vi "main.vi"() -> ()   [LabVIEW 2021]
uses:
  CTLs/msg.ctl
  <vilib>/MakerHub/LINX/Private/Type Defs/LINX Ref.ctl
  <vilib>/MakerHub/LINX/Private/Type Defs/Platform.ctl
  <vilib>/MakerHub/LINX/Private/Type Defs/Interface.ctl
  <vilib>/MakerHub/LINX/Private/Device/Type Defs/LINX Device Config.ctl
  <vilib>/MakerHub/LINX/Private/Device/Type Defs/TCP Config.ctl
  <vilib>/MakerHub/LINX/Private/Device/Type Defs/Channels.ctl
  <vilib>/MakerHub/LINX/Private/Local IO/LinxI2cWrite.vi
  <vilib>/MakerHub/LINX/Public/Utilities/Check Channel.vi
  <vilib>/MakerHub/LINX/Public/Utilities/Open Serial.vi
  <vilib>/MakerHub/LINX/Private/Utilties/Generate Error.vi
  <vilib>/Utility/error.llb/Error Cluster From Error Code.vi
  <vilib>/ErrorRing/Error Ring.xnode
  <vilib>/MakerHub/LINX/LMH-LINX.lvlib
  <vilib>/MakerHub/LINX/Private/Device/Device.lvlib
panel:
  in  "info.I2C Slave Address":u8
  in  "info.Data":u8[](array[numeric])
  in  "Serial Port":refnum<visa-resource-name>="N/A"
  in  "Error In":errorcluster
  in  "error in (no error)":errorcluster
  in  "msg":T1={"mensaje"="", "info"={"I2C Slave Address "=0, "Data"=[0]}, "LINX Resource"={"IO"=enum."Remote", "Interface"=enum."Serial", "LINX Device Config"={"Interface"=enum."Serial", "COM Port"="", "TCP Configuration"={"IP Address"="", "Port"=0}, "Device Family"=0, "Device ID"=0, "Device Name"="", "TCP Ref"=refnum, "Channels"={"DI"=[], "DO"=[], "AI"=[], "AO"=[], "PWM"=[], "QE"=[], "UART"=[], "I2C 2"=[], "SPI"=[], "CAN"=[], "Servo"=[], "AI Ref (V)"=0.0, "AI Resolution (Bits)"=0, "AO Ref (V)"=0.0, "AO Resolution (Bits)"=0}}}}
  in  "Stop":bool
  in  "Action 2":bool
  in  "Escribir":bool
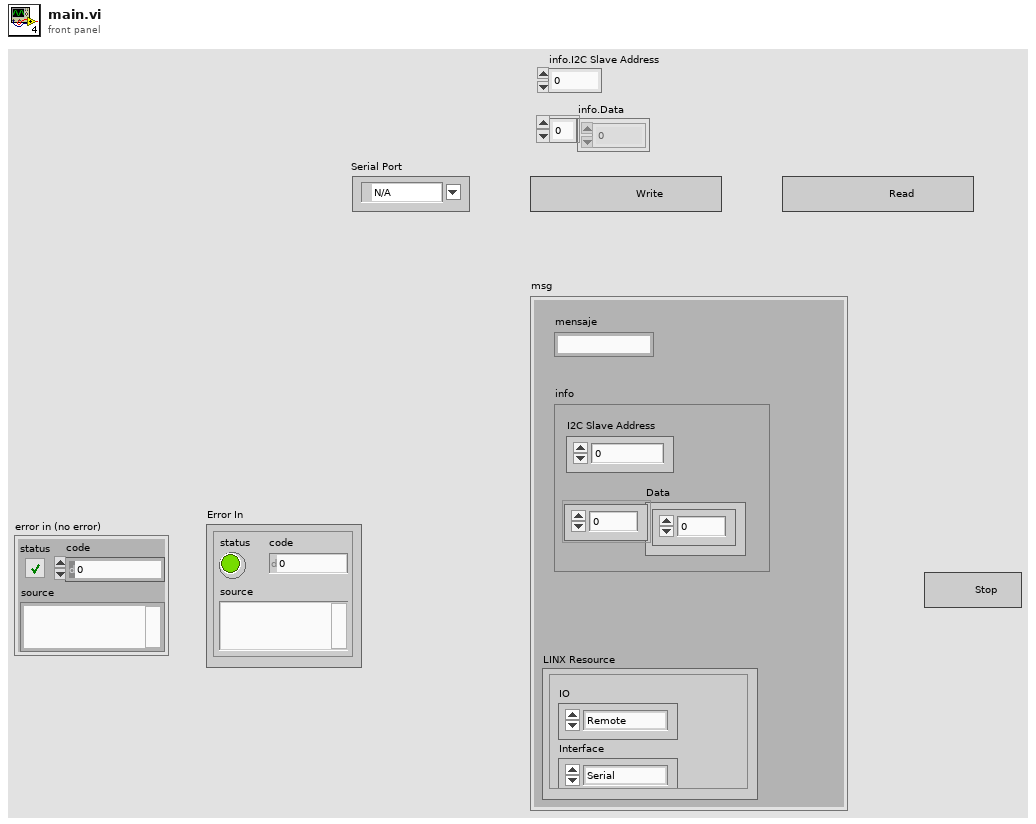
[diagram p1: front panel]
types:
  T1 = typedef "msg.ctl" = cluster{"mensaje":string, "info":cluster{"I2C Slave Address ":u8, "Data":u8[]}, "LINX Resource":T2}
  T2 = typedef "LMH-LINX.lvlib/LINX Ref.ctl" = cluster{"IO":T3, "Interface":T4, "LINX Device Config":T5}
  T3 = typedef "LMH-LINX.lvlib/Platform.ctl" = enum16{"Remote", "Local"}
  T4 = typedef "LMH-LINX.lvlib/Interface.ctl" = enum16{"Serial", "TCP"}
  T5 = typedef "LMH-LINX.lvlib/Device.lvlib/LINX Device Config.ctl" = cluster{"Interface":T4, "COM Port":refnum<visa-resource-name>, "TCP Configuration":T6, "Device Family":u8, "Device ID":u8, "Device Name":string, "TCP Ref":refnum<k5>, "Channels":T7}
  T6 = typedef "LMH-LINX.lvlib/Device.lvlib/TCP Config.ctl" = cluster{"IP Address":string, "Port":u16}
  T7 = typedef "LMH-LINX.lvlib/Channels.ctl" = cluster{"DI":u8[], "DO":u8[], "AI":u8[], "AO":u8[], "PWM":u8[], "QE":u8[], "UART":u8[], "I2C 2":u8[], "SPI":u8[], "CAN":u8[], "Servo":u8[], "AI Ref (V)":dbl, "AI Resolution (Bits)":u8, "AO Ref (V)":dbl, "AO Resolution (Bits)":u8}
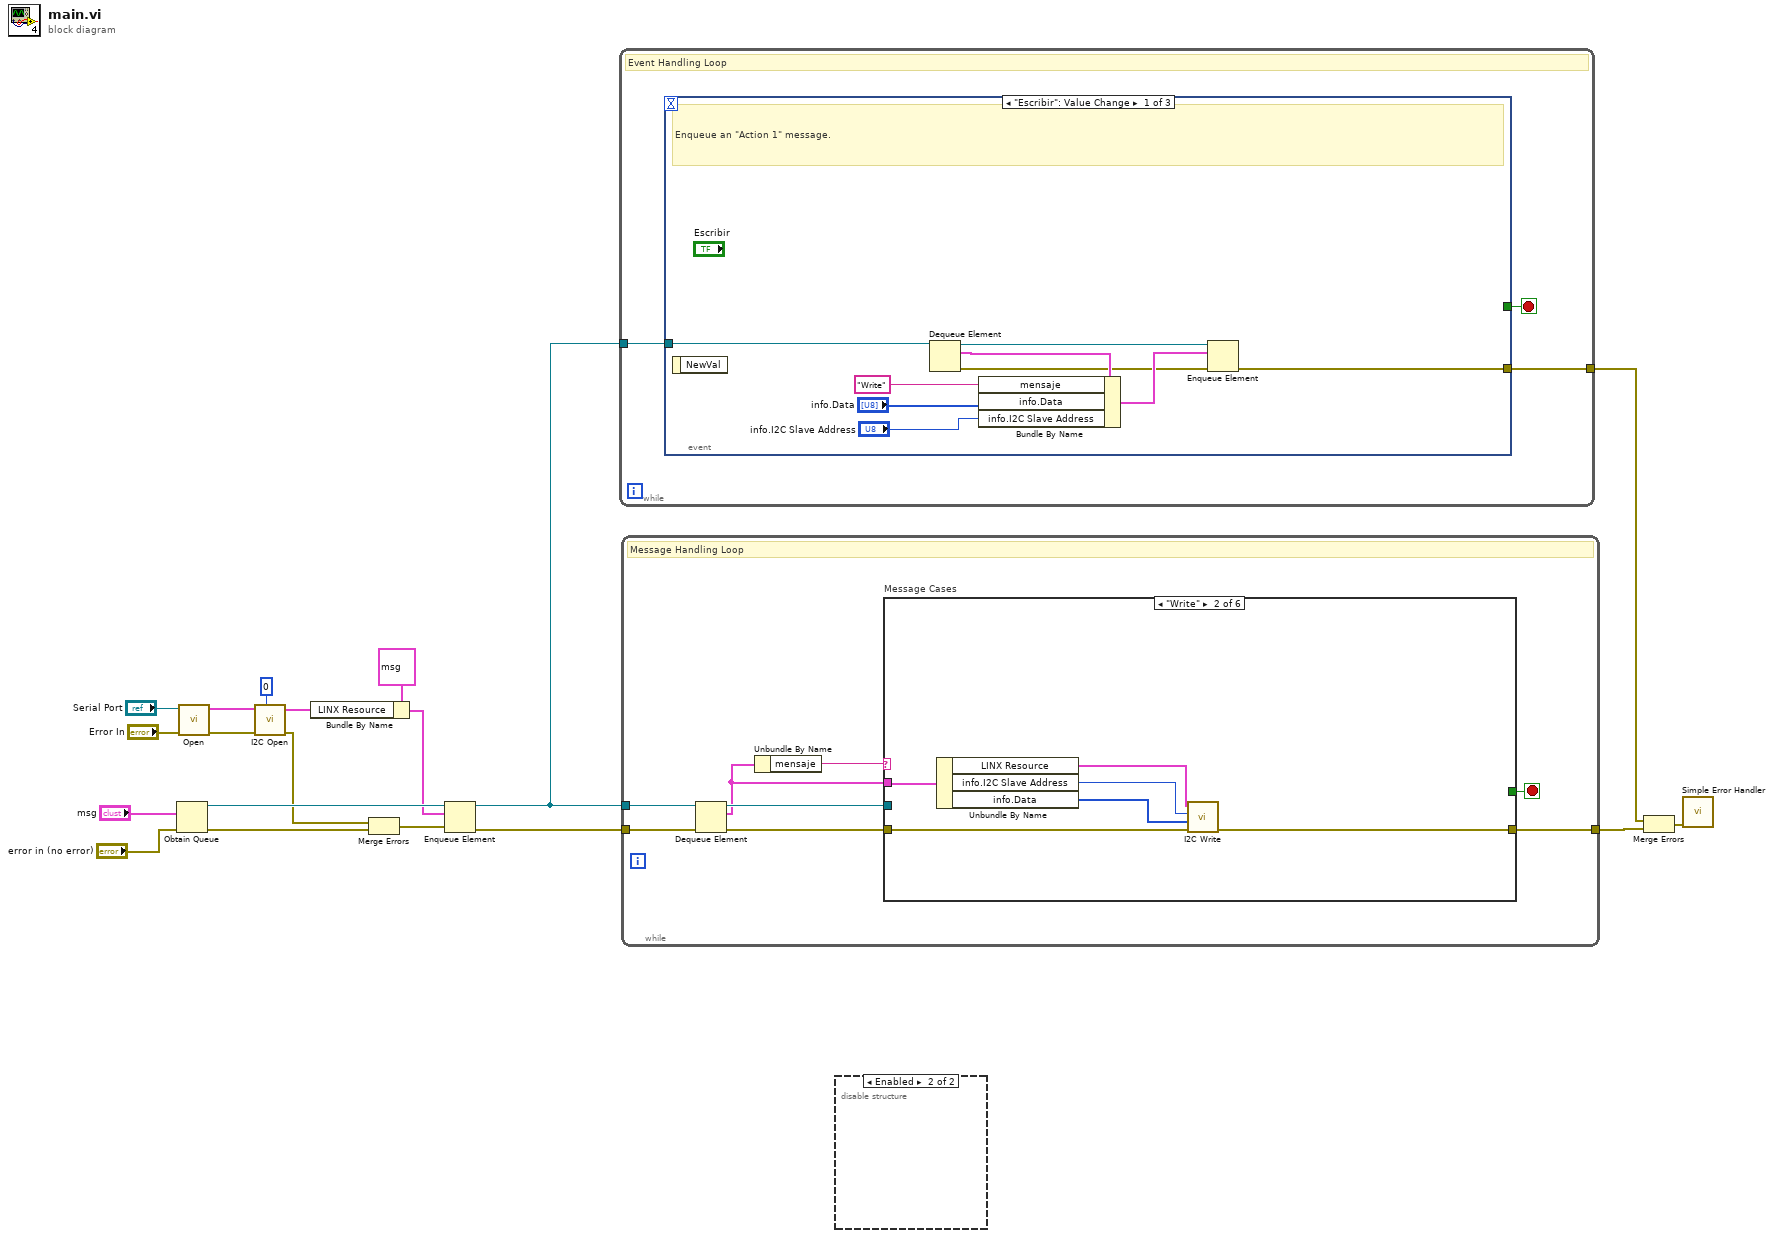
[diagram p0: block diagram]
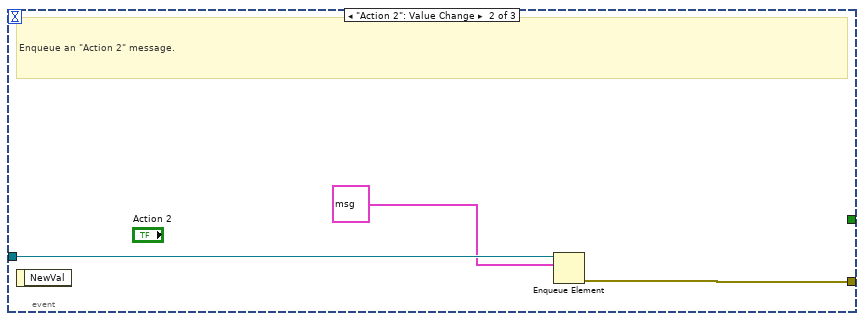
[diagram p2: hidden frame]
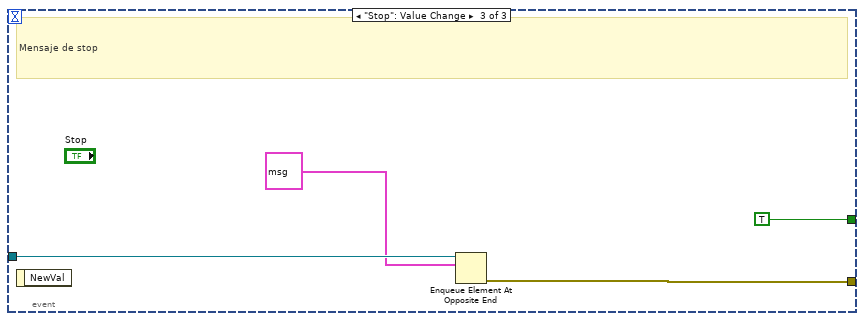
[diagram p3: hidden frame]
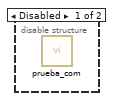
[diagram p4: hidden frame]
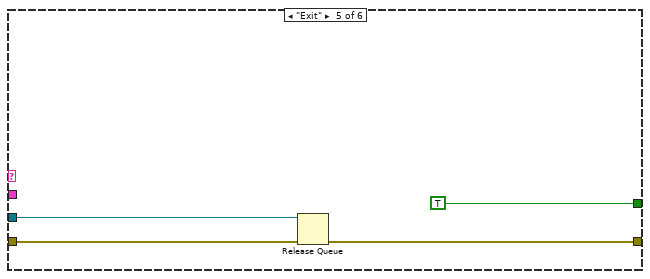
[diagram p8: hidden frame]
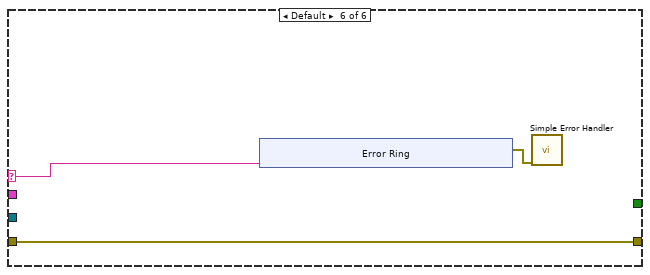
[diagram p9: hidden frame]
diagram:
  n1 = Obtain Queue(element data type="msg", error in (no error)="error in (no error)") -> (queue out=w17:refnum<queue>, error out=w6:errorcluster)  [unwired: 3 in, 1 out]
  n2 = call-poly <vilib>:"Open.vi"("Error In"="Error In", "Serial Port"="Serial Port") -> ("Error Out"=w8:errorcluster, "LINX Resource"=w9:T2)  [unwired: 7 in, 1 out]
  n3 = call <vilib>:"I2C Open.vi"("I2C Channel (0)"=u8 0, "Error In"=w8, "LINX Resource"=w9) -> ("Error Out"=w4:errorcluster, "LINX Resource"=w2:T2)  [unwired: 7 in]
  n4 = Bundle By Name(cluster=T1 {"mensaje"="Init", "info"={"I2C Slave Address "=0, "Data"=[0]}, "LINX Resource"={"IO"=enum."Remote", "Interface"=enum."Serial", "LINX Device Config"={"Interface"=enum."Serial", "COM Port"="", "TCP Configuration"={"IP Address"="", "Port"=0}, "Device Family"=0, "Device ID"=0, "Device Name"="", "TCP Ref"=refnum, "Channels"={"DI"=[], "DO"=[], "AI"=[], "AO"=[], "PWM"=[], "QE"=[], "UART"=[], "I2C 2"=[], "SPI"=[], "CAN"=[], "Servo"=[], "AI Ref (V)"=0.0, "AI Resolution (Bits)"=0, "AO Ref (V)"=0.0, "AO Resolution (Bits)"=0}}}} ("element 2"), "LINX Resource"=w2) -> (w1:T1)
  n5 = Merge Errors(w4, w6) -> (w5:errorcluster)
  n6 = Enqueue Element(queue=w17, element=w1, error in (no error)=w5) -> (queue out=w15:refnum<queue>, error out=w16:errorcluster)  [unwired: 1 in, 1 out]
  n7 = while {
    tunnel: w15 -> [w22]
    tunnel: [w20] -> w18
    stop <- w21 stop-if-true
    # "Event Handling Loop"
    n8 = event shown="[0] \"Escribir\": Value Change" {
      selector: _ -> [_ _ _]
      dyn-events: _ -> [_ _ _]
      timeout: _ -> [_ _ _]
      tunnel: [_ _ TRUE] -> w21
      tunnel: w22 -> [w30 w34 w38]
      tunnel: [w31 w33 w37] -> w20
      event "Escribir": Value Change {
        # "Enqueue an \"Action 1\" message."
        n9 = event-data() -> ()  [unwired: 1 in, 1 out]
        n10 = Dequeue Element(queue=w30) -> (queue out=w29:refnum<queue>, element=w28:T1, error out=w24:errorcluster)  [unwired: 2 in, 1 out]
        n11 = Bundle By Name(cluster=w28, "mensaje"="Write", "info.Data"="info.Data", "info.I2C Slave Address"="info.I2C Slave Address") -> (w25:T1)
        n12 = Enqueue Element(queue=w29, element=w25, error in (no error)=w24) -> (error out=w31:errorcluster)  [unwired: 1 in, 2 out]
      }
      event "Action 2": Value Change {
        # "Enqueue an \"Action 2\" message."
        n13 = event-data() -> ()  [unwired: 1 in, 1 out]
        n14 = Enqueue Element(queue=w34, element=T1 {"mensaje"="Read", "info"={"I2C Slave Address "=0, "Data"=[0]}, "LINX Resource"={"IO"=enum."Remote", "Interface"=enum."Serial", "LINX Device Config"={"Interface"=enum."Serial", "COM Port"="", "TCP Configuration"={"IP Address"="", "Port"=0}, "Device Family"=0, "Device ID"=0, "Device Name"="", "TCP Ref"=refnum, "Channels"={"DI"=[], "DO"=[], "AI"=[], "AO"=[], "PWM"=[], "QE"=[], "UART"=[], "I2C 2"=[], "SPI"=[], "CAN"=[], "Servo"=[], "AI Ref (V)"=0.0, "AI Resolution (Bits)"=0, "AO Ref (V)"=0.0, "AO Resolution (Bits)"=0}}}}) -> (error out=w33:errorcluster)  [unwired: 2 in, 2 out]
      }
      event "Stop": Value Change {
        # "Mensaje de stop"
        n15 = event-data() -> ()  [unwired: 1 in, 1 out]
        n16 = Enqueue Element At Opposite End(queue=w38, element=T1 {"mensaje"="Exit", "info"={"I2C Slave Address "=0, "Data"=[0]}, "LINX Resource"={"IO"=enum."Remote", "Interface"=enum."Serial", "LINX Device Config"={"Interface"=enum."Serial", "COM Port"="", "TCP Configuration"={"IP Address"="", "Port"=0}, "Device Family"=0, "Device ID"=0, "Device Name"="", "TCP Ref"=refnum, "Channels"={"DI"=[], "DO"=[], "AI"=[], "AO"=[], "PWM"=[], "QE"=[], "UART"=[], "I2C 2"=[], "SPI"=[], "CAN"=[], "Servo"=[], "AI Ref (V)"=0.0, "AI Resolution (Bits)"=0, "AO Ref (V)"=0.0, "AO Resolution (Bits)"=0}}}}) -> (error out=w37:errorcluster)  [unwired: 2 in, 2 out]
      }
    }
  }
  n17 = while {
    tunnel: w15 -> [w43]
    tunnel: w16 -> [w44]
    tunnel: [w45] -> w19
    stop <- w46 stop-if-true
    # "Message Handling Loop"
    n18 = Dequeue Element(queue=w43, error in (no error)=w44) -> (queue out=w42:refnum<queue>, element=w39:T1, error out=w41:errorcluster)  [unwired: 1 in, 1 out]
    n19 = Unbundle By Name(w39) -> ("mensaje"=w40:string)
    n20 = case "Message Cases" shown="\"Write\"" w40 {
      selector: w40 -> [_ _ _ _ _ w62]
      tunnel: w42 -> [_ _ _ _ w59 _]
      tunnel: w41 -> [w47 w53 w54 w55 w57 w61]
      tunnel: [w47 w52 w54 w55 w56 w61] -> w45
      tunnel: [_ _ _ _ TRUE _] -> w46
      tunnel: w39 -> [_ w51 _ _ _ _]
      frame "Init" {
        # "Initialize - Perform any initialization code for your application here. In this example, the only initialization required is setting the Display Message indicator value to an empty string."
      }
      frame "Write" {
        # "Action 1 - Send an \"Update Display\" message indicating which button was pressed. Note that a string is sent as the Message Data along with the \"Update Display\" message."
        n21 = Unbundle By Name(w51) -> ("LINX Resource"=w50:T2, "info.I2C Slave Address"=w49:u8, "info.Data"=w48:u8[])
        n22 = call <vilib>:"I2C Write.vi"("Error In"=w53, "Data"=w48, "I2C Slave Address (0)"=w49, "LINX Resource"=w50) -> ("Error Out"=w52:errorcluster)  [unwired: 6 in, 1 out]
      }
      frame "Read" {
        # "sdff"
      }
      frame "Update Display" {
        # "Update Display - Convert the Message Data to a string to display in the Display Message indicator."
      }
      frame "Exit" {
        # "Exit - Exit the application. Since this message was sent as a priority message (i.e., it was placed at the front of the queue), any cleanup code should run here, since the loop is about to stop. Any other messages in the queue will not be handled."
        n23 = Release Queue(queue=w59, error in (no error)=w57) -> (error out=w56:errorcluster)  [unwired: 1 in, 2 out]
      }
      frame Default {
        # "The Default case only runs if there is a message that isn't defined in any of the other cases. Generate an error if this occurs."
        n24 = xnode "Error Ring"("parameter 0"=w62) -> ("error out"=w60:errorcluster)
        n25 = call <vilib>:"Simple Error Handler.vi"("error in (no error)"=w60) -> ()  [unwired: 4 in, 5 out]
      }
    }
  }
  n26 = disable-structure shown="Enabled" {
    frame Disabled {
      n27 = call "prueba_com.vi"() -> ()  [unwired: 12 in]
    }
    frame Enabled {
    }
  }
  n28 = Merge Errors(w18, w19) -> (w14:errorcluster)
  n29 = call <vilib>:"Simple Error Handler.vi"("error in (no error)"=w14) -> ()  [unwired: 4 in, 5 out]
